vi "Create Events.vi"(7 "error in":errorcluster, 10 "Message Pump in":refnum<class "Message Pump.lvclass">) -> (0 "error out":errorcluster, 2 "Event Registration Refnum":refnum<event-registration>, 3 "Message Pump out":refnum<class "Message Pump.lvclass">)   [LabVIEW 2023, in "Message Pump.lvclass"]
uses:
  Message Pump.lvclass
  <vilib>/addons/_Workers/Library/Case Label.ctl
  <vilib>/addons/_Workers/Library/Classes/Message Queue/Message Queue.lvclass
  Message Pump.lvclass/Message Pump.ctl
  <vilib>/addons/_Workers/Library/Workers.lvlib
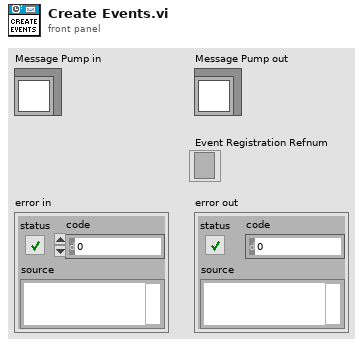
[diagram p1: front panel]
types:
  T1 = typedef "WORKERS.lvlib/Case Label.ctl" = string
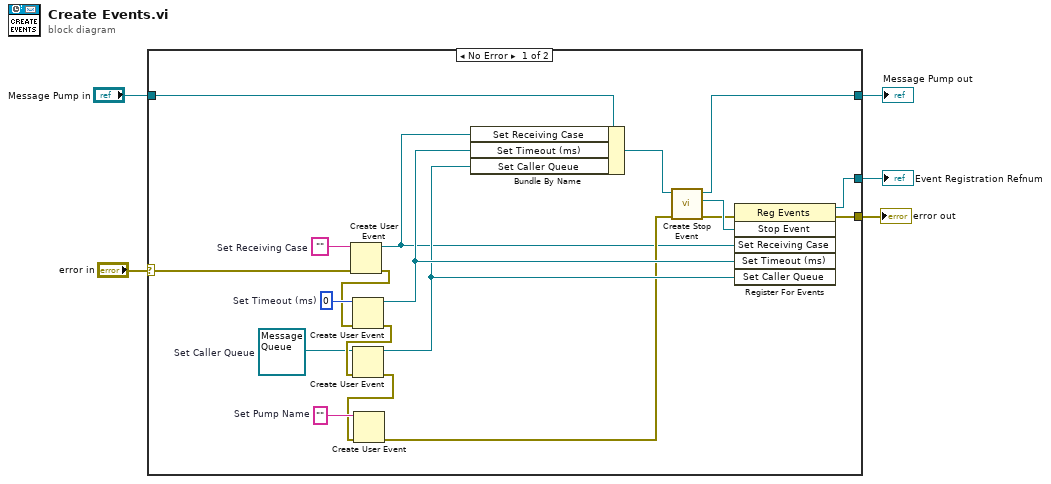
[diagram p0: block diagram]
diagram:
  n1 = case shown="No Error" "error in" {
    selector: "error in" -> [w13 w26]
    tunnel: [w24 w26] -> w5
    tunnel: [w20 _] -> w1
    tunnel: "Message Pump in" -> [w16 w25]
    tunnel: [w17 w25] -> w2
    frame No Error {
      w6 = T1 ""  # Set Receiving Case
      w10 = ""  # Set Pump Name
      w12 = refnum<class "Message Queue.lvclass"> refnum  # Set Caller Queue
      w22 = 0  # Set Timeout (ms)
      n2 = Create User Event(user event datatype=w6, error in=w13) -> (user event=w7:refnum<user-event>, error out=w14:errorcluster)
      n3 = Create User Event(user event datatype=w22, error in=w14) -> (user event=w23:refnum<user-event>, error out=w21:errorcluster)
      n4 = Create User Event(user event datatype=w12, error in=w21) -> (user event=w11:refnum<user-event>, error out=w9:errorcluster)
      n5 = Create User Event(user event datatype=w10, error in=w9) -> (error out=w8:errorcluster)  [unwired: 1 out]
      n6 = Bundle By Name(cluster=w16, "Set Receiving Case"=w7, "Set Timeout (ms)"=w23, "Set Caller Queue"=w11) -> (w15:refnum<class "Message Pump.lvclass">)
      n7 = call-dynamic "Create Stop Event.vi"("error in"=w8, "Worker"=w15) -> ("error out"=w18:errorcluster, "Stop Event"=w19:refnum<user-event>, "Worker out"=w17:refnum<class "Message Pump.lvclass">)  [unwired: 7 in]
      n8 = register-events(error in=w18, w19, w7, w23, w11) -> (reference out=w20:refnum<event-registration>, error out=w24:errorcluster)  [unwired: 1 in]
    }
    frame Error {
    }
  }
  "error out" <- w5
  "Message Pump out" <- w2
  "Event Registration Refnum" <- w1
